vi "SPD.HV_Bias setup.vi"(5 "Graph":refnum<vi>, 7 "Progress":refnum<vi>, 8 "Error In":errorcluster, 11 "SPD.Stand Ctrl in":T1 {"spdDeviceSession"."hidSPD.Controller"."HV_bias" format="%#_6p, V"; "spdDeviceSession"."hidSPD.Controller"."TSet" format="%#_6p, DegC"}) -> (0 "Error Out":errorcluster, 1 "pass":bool, 2 "result":string, 3 "SPD.Stand Ctrl out":T1 {"spdDeviceSession"."hidSPD.Controller"."HV_bias" format="%#_6p, V"; "spdDeviceSession"."hidSPD.Controller"."TSet" format="%#_6p, DegC"})   [LabVIEW 2018]
uses:
  typedefs/SPD.Stand Ctrl.ctl
  Instruments/SPD HID Interface/hidSPDLibForLabView/LibVIs/hidSPD Controls/hidSPD Device Session.ctl
  Instruments/SPD HID Interface/hidSPDLibForLabView/LibVIs/hidSPD Controls/hidSPD Controller.ctl
  Instruments/KC705 DevBoard/typedefs/DevB.Session.ctl
  Instruments/KeySight 53230A/typedefs/FreqC.Session.ctl
  Instruments/KeySight 8164B/KeySight 8164B LAN InstrLib/typedefs/KeySight 8164B control.ctl
  Instruments/LeCroy SDA830/typedefs/LeCroy.Session.ctl
  typedefs/SPD.Events.ctl
  <vilib>/Utility/config.llb/Config Data RefNum.ctl
  typedefs/SPD.Meas Result.ctl
  SubVIs/Min_Max.ctl
  SubTests/01_HV_Bias Test/SPD.HV_Bias Test Limits.vi
  SubVIs/comparison mode.ctl
  Instruments/KeySight 8164B/KeySight 8164B LAN InstrLib.lvlib
  Instruments/SPD HID Interface/hidSPDLibForLabView/hidSPDLibForLabView.lvlib
  <vilib>/Utility/config.llb/NI_LVConfig.lvlib
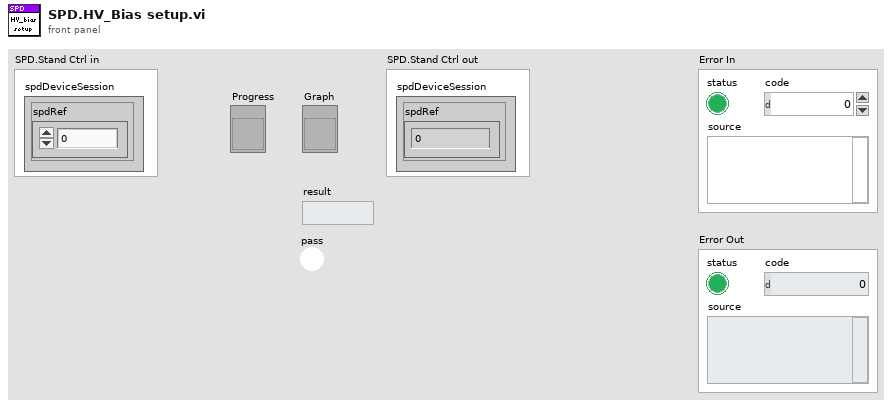
[diagram p1: front panel]
types:
  T1 = typedef "SPD.Stand Ctrl.ctl" = cluster{"spdDeviceSession":T2, "DevBSession":T4, "FreqCSession":T5, "8164BSession":T6, "LeCroySession":T7, "Events":T8, "configFile":T9, "SPD.Result":T10}
  T2 = typedef "hidSPDLibForLabView.lvlib/hidSPD Device Session.ctl" = cluster{"spdRef":u64, "connected":bool, "spdName":string, "hidSPD.Controller":T3}
  T3 = typedef "hidSPDLibForLabView.lvlib/hidSPD Controller.ctl" = cluster{"TSet":sgl, "HV_bias":sgl, "DDS_stb_code":u16}
  T4 = typedef "DevB.Session.ctl" = cluster{"DevBRef":refnum<visa-resource-name>, "connected":bool}
  T5 = typedef "FreqC.Session.ctl" = cluster{"FreqCRef":refnum<visa-resource-name>, "timeout":dbl, "connected":bool}
  T6 = typedef "KeySight 8164B LAN InstrLib.lvlib/KeySight 8164B control.ctl" = cluster{"Connection ID":refnum<k5>, "Connected":bool, "Info":string, "Slots Info":string[]}
  T7 = typedef "LeCroy.Session.ctl" = cluster{"LeCroySession":refnum<visa-resource-name>, "connected":bool}
  T8 = typedef "SPD.Events.ctl" = cluster{"DCRTest":refnum<user-event>, "Stop":refnum<user-event>}
  T9 = typedef "NI_LVConfig.lvlib/Config Data RefNum.ctl" = refnum<k1>
  T10 = typedef "SPD.Meas Result.ctl" = cluster{"HV_Bias":dbl[], "Stb_code":dbl[], "Temprature":dbl[], "Data":dbl[][][][]}
  T11 = typedef "comparison mode.ctl" = enum16{"in range", "bigger then min", "bigger then max", "less then min", "less then max"}
  T12 = typedef "SPD.HV_Bias Test Limits.vi" = cluster{"start value":dbl, "stop value":dbl, "step":dbl, "gate":dbl, "num of tests":dbl, "range":T13, "comparison mode":T11}
  T13 = typedef "Min_Max.ctl" = cluster{"min":dbl, "max":dbl}
  T14 = typedef "SPD.HV_Bias Test Params.vi" = cluster{"FS":i32, "TS":i32, "Step_Quick":dbl, "Stop_Quick":dbl, "Start_Quick":dbl, "Gate_Quick":dbl, "Step_Precise":dbl, "Gate_Precise":dbl, "max":dbl, "min":dbl}
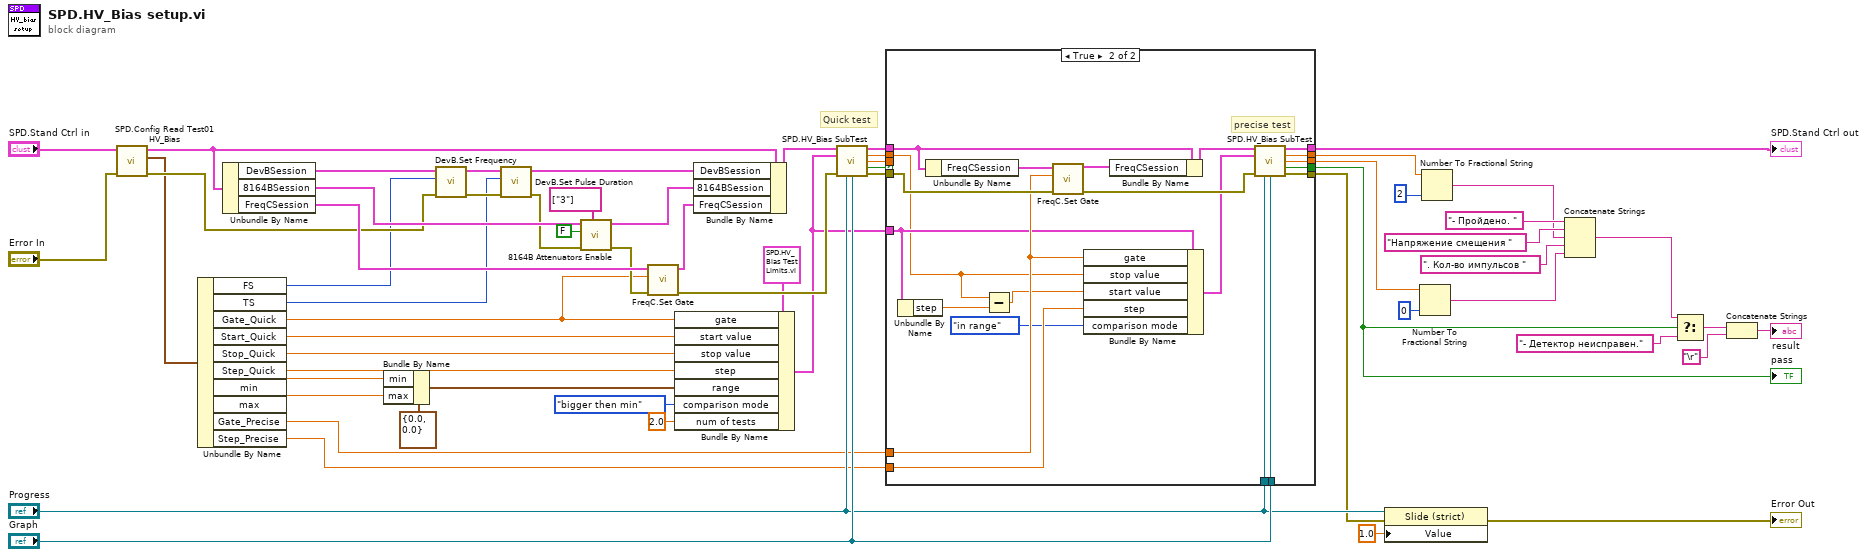
[diagram p0: block diagram]
diagram:
  # "Quick test"
  n1 = call "SPD.Config Read Test01 HV_Bias.vi"("Error In"="Error In", "SPD.Stand Ctrl in"="SPD.Stand Ctrl in") -> ("Error Out"=w32:errorcluster, "HV_TestParams"=w29:T14, "SPD.Stand Ctrl out"=w34:T1)  [unwired: 7 in]
  n2 = Unbundle By Name(w29) -> ("FS"=w28:i32, "TS"=w27:i32, "Gate_Quick"=w7:dbl, "Start_Quick"=w10:dbl, "Stop_Quick"=w9:dbl, "Step_Quick"=w8:dbl, "min"=w25:dbl, "max"=w24:dbl, "Gate_Precise"=w4:dbl, "Step_Precise"=w1:dbl)
  n3 = Unbundle By Name(w34) -> ("DevBSession"=w40:T4, "8164BSession"=w55:T6, "FreqCSession"=w54:T5)
  n4 = Bundle By Name(cluster=T13 {"min"=0.0, "max"=0.0} ("minMax"), "min"=w25, "max"=w24) -> (w6:T13)
  n5 = call "DevB.Set Frequency.vi"("error in (no error)"=w32, "Frequency"=w28, "DevB Session in"=w40) -> ("error out"=w41:errorcluster, "DevB Session out"=w42:T4)  [unwired: 7 in]
  n6 = call "DevB.Set Pulse Duration.vi"("error in (no error)"=w41, "Pulse Duration"=w27, "DevB Session in"=w42) -> ("error out"=w38:errorcluster, "DevB Session out"=w39:T4)  [unwired: 7 in]
  n7 = call "8164B Attenuators Enable.vi"("Slots"=string[] ["3"], "error in"=w38, "Enable"=FALSE, "KeySight 8164B control in"=w55) -> ("error out"=w53:errorcluster, "KeySight 8164B control out"=w52:T6)  [unwired: 6 in]
  n8 = call "FreqC.Set Gate.vi"("error In"=w53, "Gate, sec"=w7, "FreqC Session in"=w54) -> ("error out"=w30:errorcluster, "FreqC Session out"=w51:T5)  [unwired: 7 in]
  n9 = Bundle By Name(cluster=T12 {"start value"=0.0, "stop value"=0.0, "step"=0.0, "gate"=0.0, "num of tests"=0.0, "range"={"min"=0.0, "max"=0.0}, "comparison mode"=enum."in range"} ("SPD.HV_bias Test Limits"), "gate"=w7, "start value"=w10, "stop value"=w9, "step"=w8, "range"=w6, "comparison mode"=comparison_mode."bigger then min", "num of tests"=2.0) -> (w3:T12)
  n10 = Bundle By Name(cluster=w34, "DevBSession"=w39, "8164BSession"=w52, "FreqCSession"=w51) -> (w31:T1)
  n11 = call "SPD.HV_Bias SubTest.vi"("SPD.Stand Ctrl in"=w31, "SPD.HV_bias Test Limits"=w3, "Error In"=w30, "Progress"="Progress", "Graph"="Graph") -> ("SPD.Stand Ctrl out"=w22:T1, "last HV_bias"=w20:dbl, "Clicks Count"=w12:dbl, "result"=w14:bool, "Error Out"=w21:errorcluster)  [unwired: 6 in]
  n12 = case shown="True" w14 {
    selector: w14 -> [w65 _]
    tunnel: "Graph" -> [_ w87]
    tunnel: w4 -> [_ w73]
    tunnel: w22 -> [w66 w85]
    tunnel: w21 -> [w64 w83]
    tunnel: w20 -> [w63 w70]
    tunnel: "Progress" -> [_ w81]
    tunnel: [w64 w80] -> w18
    tunnel: [w66 w78] -> w17
    tunnel: [w63 w77] -> w16
    tunnel: [w62 w76] -> w15
    tunnel: [w65 w75] -> w13
    tunnel: w12 -> [w62 _]
    tunnel: w3 -> [_ w72]
    tunnel: w1 -> [_ w68]
    frame False {
    }
    frame True {
      # "precise test"
      n13 = Unbundle By Name(w72) -> ("step"=w71:dbl)
      n14 = Unbundle By Name(w85) -> ("FreqCSession"=w86:T5)
      n15 = Subtract(x=w70, y=w71) -> (x-y=w69:dbl)
      n16 = call "FreqC.Set Gate.vi"("error In"=w83, "Gate, sec"=w73, "FreqC Session in"=w86) -> ("error out"=w79:errorcluster, "FreqC Session out"=w84:T5)  [unwired: 7 in]
      n17 = Bundle By Name(cluster=w72, "gate"=w73, "stop value"=w70, "start value"=w69, "step"=w68, "comparison mode"=comparison_mode."in range" ("Comparison Mode")) -> (w74:T12)
      n18 = Bundle By Name(cluster=w85, "FreqCSession"=w84) -> (w82:T1)
      n19 = call "SPD.HV_Bias SubTest.vi"("SPD.Stand Ctrl in"=w82, "SPD.HV_bias Test Limits"=w74, "Error In"=w79, "Progress"=w81, "Graph"=w87) -> ("SPD.Stand Ctrl out"=w78:T1, "last HV_bias"=w77:dbl, "Clicks Count"=w76:dbl, "result"=w75:bool, "Error Out"=w80:errorcluster)  [unwired: 6 in]
    }
  }
  "SPD.Stand Ctrl out" <- w17
  "pass" <- w13
  n20 = property class="Slide (strict)"(reference="Progress", error in=w18, "Value"=1.0) -> (error out=→"Error Out":errorcluster)  [unwired: 1 out]
  n21 = Number To Fractional String(number=w15, precision (6)=i16 0) -> (F-format string=w44:string)  [unwired: 2 in]
  n22 = Number To Fractional String(number=w16, precision (6)=i16 2) -> (F-format string=w47:string)  [unwired: 2 in]
  n23 = Concatenate Strings("- Пройдено. " ("report"), "Напряжение смещения " ("report"), w47, ". Кол-во импульсов " ("report"), w44) -> (w50:string)
  n24 = Select(t=w50, s=w13, f="- Детектор неисправен.") -> (s? t:f=w59:string)
  n25 = Concatenate Strings(w59, "\r") -> (→"result":string)
